vi "NavGPSmap.vi"() -> ()   [LabVIEW 2009]
uses:
  TypeDefs/Sensor TypeDefs/GPS Data.ctl
  <vilib>/picture/cartesn2.llb/XY Plot Type.ctl
panel:
  out "XY Graph 2":cluster{"Y":dbl[], "Y":dbl[]}[](graph)
  in  "stop 2":bool
  in  "XY plot cosmetics 2":T2={"plot color"=16776960, "XY plot type"=enum."connected points", "baseline"=0.0} {"baseline" format="%0.2f"}
  in  "[sized scatter plot cosmetics]":T3={"min size"=1, "max size"=5, "maps to max size"=5, "color array"=[16776960, 65280, 16711680, 255]}
  in  "XY plot cosmetics":T2={"plot color"=16776960, "XY plot type"=enum."connected points", "baseline"=0.0} {"baseline" format="%0.2f"}
  in  "cartesian grid cosmetics":T4={"line color"=6710886, "text color"=13421772, "tick length(3)"=3, "crossing axes"=FALSE, "visible grid?"=TRUE}
  in  "cartesian axis attributes":T5={"x minimum"=0.0, "x maximum"=0.0, "x log?"=FALSE, "x precision"=1, "x format"=enum."Decimal", "y minimum"=0.0, "y maximum"=0.0, "y log?"=FALSE, "y precision"=1, "y format"=enum."Decimal"} {"x minimum" format="%0.2f"; "x maximum" format="%0.2f"; "y minimum" format="%0.2f"; "y maximum" format="%0.2f"}
  in  "stop":bool
  in  "WP List":T6[](array[typedef]) {"Longitude" format="%#_14g"; "Latitude" format="%#_14g"}
  out "new picture":picture
  in  "Current Co-ordinates":T6 {"Longitude" format="%#_14g"; "Latitude" format="%#_14g"}
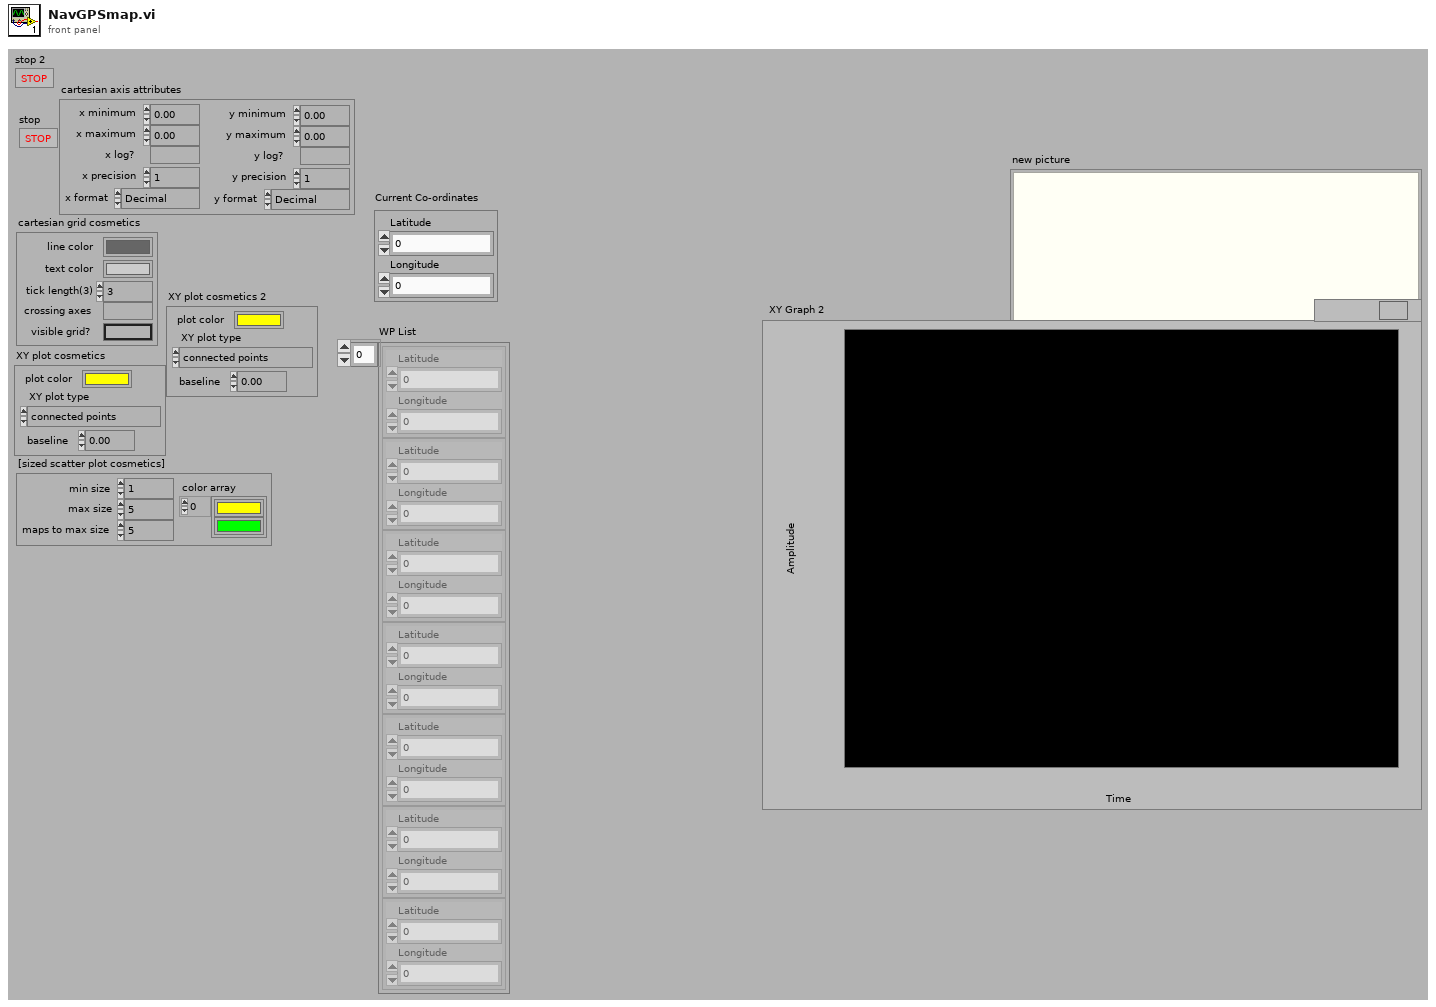
[diagram p1: front panel]
types:
  T1 = typedef "XY Plot Type.ctl" = enum16{"points", "squares", "circles", "connected points", "connected squares", "connected circles", "comb plot", "sized scatter plot", "sized-colored scatter plot", "min-max lines"}
  T2 = cluster{"plot color":u32, "XY plot type":T1, "baseline":dbl}
  T3 = cluster{"min size":i16, "max size":i16, "maps to max size":i16, "color array":u32[]}
  T4 = cluster{"line color":u32, "text color":u32, "tick length(3)":i16, "crossing axes":bool, "visible grid?":bool}
  T5 = cluster{"x minimum":dbl, "x maximum":dbl, "x log?":bool, "x precision":u8, "x format":enum8{"Decimal", "Scientific", "Engineering", "Binary", "Octal", "Hex"}, "y minimum":dbl, "y maximum":dbl, "y log?":bool, "y precision":u8, "y format":enum8{"Decimal", "Scientific", "Engineering", "Binary", "Octal", "Hex"}}
  T6 = typedef "GPS Data.ctl" = cluster{"Latitude":dbl, "Longitude":dbl}
  T7 = cluster{"WP List[0]":T6, "WP List[1]":T6, "WP List[2]":T6, "WP List[3]":T6, "WP List[4]":T6, "WP List[5]":T6, "WP List[6]":T6, "WP List[7]":T6, "WP List[8]":T6}
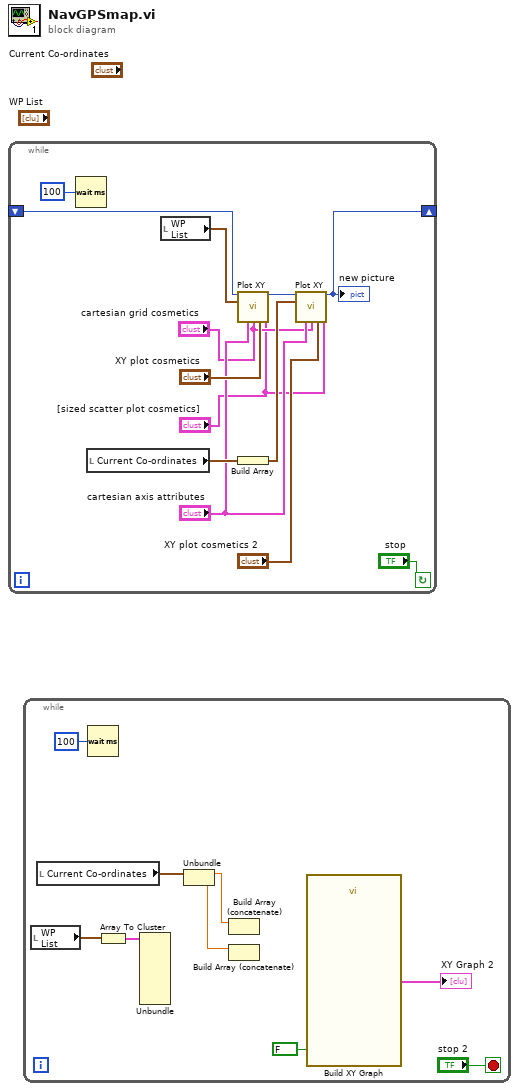
[diagram p0: block diagram]
diagram:
  n1 = while {
    shift-right: [w7] -> _
    shift-left: _ -> [w13]
    stop <- "stop" continue-if-true
    n2 = Wait (ms)(milliseconds to wait=u32 100) -> ()  [unwired: 1 out]
    n3 = local read "Current Co-ordinates"() -> (w10:T6)
    n4 = local read "WP List"() -> (w12:T6[])
    n5 = call <vilib>:"Plot XY.vi"("picture"=w13, "data"=w12, "cartesian axis attributes"="cartesian axis attributes", "cartesian grid cosmetics"="cartesian grid cosmetics", "XY plot cosmetics"="XY plot cosmetics", "[sized scatter plot cosmetics]"="[sized scatter plot cosmetics]") -> ("new picture"=w11:picture)  [unwired: 9 in]
    n6 = Build Array(w10) -> (w9:T6[])
    n7 = call <vilib>:"Plot XY.vi"("picture"=w11, "data"=w9, "cartesian axis attributes"="cartesian axis attributes", "cartesian grid cosmetics"="cartesian grid cosmetics", "XY plot cosmetics"="XY plot cosmetics 2", "[sized scatter plot cosmetics]"="[sized scatter plot cosmetics]") -> ("new picture"=w7:picture)  [unwired: 9 in]
    "new picture" <- w7
  }
  n8 = while {
    stop <- "stop 2" stop-if-true
    n9 = local read "WP List"() -> (w15:T6[])
    n10 = local read "Current Co-ordinates"() -> (w19:T6)
    n11 = Wait (ms)(milliseconds to wait=u32 100) -> ()  [unwired: 1 out]
    n12 = Array To Cluster(array=w15) -> (cluster=w14:T7)
    n13 = Unbundle(w14) -> ()  [unwired: 9 out]
    n14 = Unbundle(w19) -> ("Latitude"=w17:dbl, "Longitude"=w16:dbl)
    n15 = Build Array (concatenate)(w17) -> ()  [unwired: 1 in, 1 out]
    n16 = Build Array (concatenate)(w16) -> ()  [unwired: 1 in, 1 out]
    n17 = call "Build XY Graph"("Reset"=FALSE) -> ("XY Graph"=→"XY Graph 2":cluster{"Y":dbl[], "Y":dbl[]}[])  [unwired: 9 in, 1 out]
  }
